vi "FindChangedOutput.vi"(8 "StoredDigitalOutput":u8[](array[numeric]), 9 "ListOfSlotsAndOutputs":u8[](array[numeric]), 10 "MockDigitalOutput":cluster{"BufferUpdateFIFO":refnum<k21>}={"BufferUpdateFIFO"="MockDigitalOutputCommand"}, 11 "NewDigitalOutput":u8[](array[numeric])) -> (0 "NewStoredDigitalOutput":u8[](array[numeric]))   [LabVIEW 2016, in "FPGAMockDigitalOutput.lvlib"]
uses:
  FPGAMockDigitalOutput.lvlib
  <vilib>/rvi/DataTransferAndStorage/Container/Common/niFpgaContainerExecOnDevCompGetState.vi
  <vilib>/rvi/Emulation/niFpgaEmulationIsFPGAContextNoSignature.vi
  <vilib>/rvi/Emulation/niFpgaSctlEmulationGetInTimedLoop.vi
  <vilib>/rvi/errors/niFpgaSetErrorForExecOnDevCompSimple.vi
  <vilib>/rvi/eio/common/nirviEmuReportErrorAndStop.vi
  <vilib>/rvi/DataTransferAndStorage/Container/Common/niFpgaContainerGetUniqueNameForEmu.vi
  <vilib>/rvi/FIFO/Fifo_Resource/nirvififoEmulationSetSize.vi
  <vilib>/rvi/FIFO/Fifo_Resource/nirviFifoEmulationQueueMgr.vi
  <instcachedir>/0/nirviFifoEmulationQueueMgr_E5CAEC123FF24DC58D834DCA3CDAA9B5.lvgen/nirviFifoEmulationQueueMgr_E5CAEC123FF24DC58D834DCA3CDAA9B5_000.vi
  <vilib>/rvi/FIFO/Fifo_Resource/nirvififoEmulationDetermineInputValidOut.vi
  <vilib>/rvi/FIFO/Fifo_Resource/nirvififoEmulationCreateLock.vi
  <vilib>/rvi/Emulation/niFpgaProcessEmulError.vi
  <vilib>/rvi/FIFO/Fifo_Resource/nirvififoEmulationObtainLock.vi
  <vilib>/rvi/FIFO/Fifo_Resource/nirvififoEmulationReleaseLock.vi
  <vilib>/rvi/occurrence/nirviWaitOnOccurrenceBase.vi
  <vilib>/rvi/errors/nirviReportUnexpectedCaseInternalError.vi
  <vilib>/rvi/errors/nirviReportUnexpectedCaseInternalError (U32).vi
  <vilib>/Utility/error.llb/Clear Errors.vi
  <vilib>/rvi/interface/RandomDataEmulation/niFpgaRandomDataHandleErrors.vi
  <vilib>/rvi/DataTransferAndStorage/Container/XNode/niFpgaContainer.xnode
  <vilib>/rvi/FIFO/Fifo_Resource/niFpgaFifoEmulationRefIn.vi
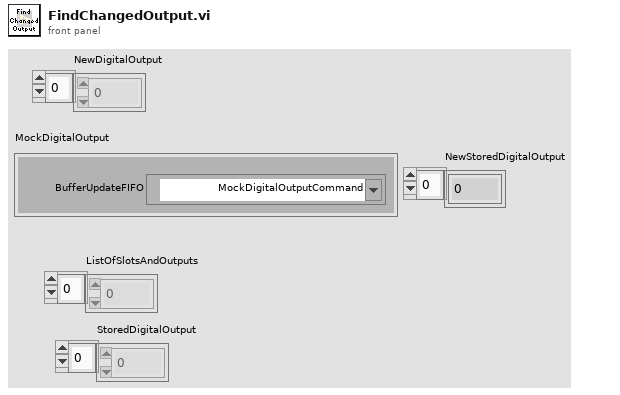
[diagram p1: front panel]
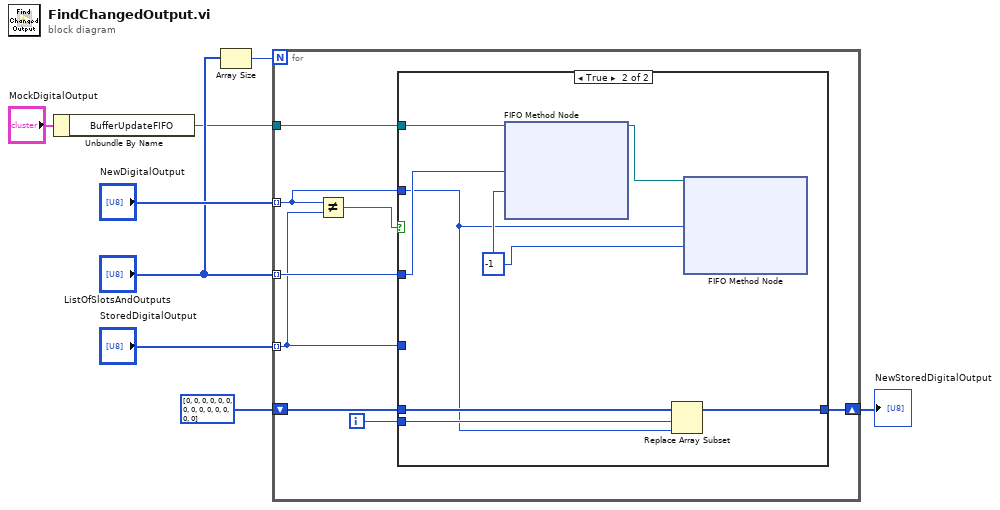
[diagram p0: block diagram]
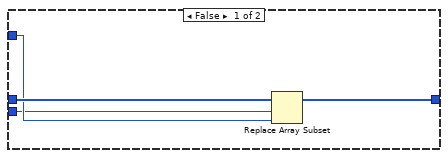
[diagram p2: hidden frame]
diagram:
  n1 = Unbundle By Name("MockDigitalOutput") -> ("BufferUpdateFIFO"=w1:refnum<k21>)
  n2 = Array Size(array="ListOfSlotsAndOutputs") -> (size(s)=w4:i32)
  n3 = for {
    N: w4 -> [_]
    tunnel: "NewDigitalOutput" -> [w14] mode=indexing
    tunnel: "ListOfSlotsAndOutputs" -> [w15] mode=indexing
    tunnel: "StoredDigitalOutput" -> [w11] mode=indexing
    shift-right: [w12] -> w5
    shift-left: u8[] [0, 0, 0, 0, 0, 0, 0, 0, 0, 0, 0, 0, 0, 0] -> [w13]
    tunnel: w1 -> [w9]
    i -> [w10]
    n4 = Not Equal?(x=w14, y=w11) -> (x != y?=w16:bool)
    n5 = case shown="True" w16 {
      tunnel: w15 -> [_ w22]
      tunnel: w14 -> [_ w21]
      tunnel: w13 -> [w20 w28]
      tunnel: [w19 w27] -> w12
      tunnel: w11 -> [w18 _]
      tunnel: w10 -> [w17 w26]
      tunnel: w9 -> [_ w25]
      frame False {
        n6 = Replace Array Subset(array=w20, new element=w18, index=w17) -> (w19:u8[])
      }
      frame True {
        w23 = -1 ("Timeout")
        n7 = xnode ("FIFO Method Node")("Element"=w22, "Timeout"=w23, "FIFO In"=w25) -> ("FIFO Out"=w24:refnum<k21>)  [unwired: 1 out]
        n8 = Replace Array Subset(array=w28, new element=w21, index=w26) -> (w27:u8[])
        n9 = xnode ("FIFO Method Node")("Element"=w21, "Timeout"=w23, "FIFO In"=w24) -> ()  [unwired: 2 out]
      }
    }
  }
  "NewStoredDigitalOutput" <- w5
